vi "FileStream_Create.vi"(7 "mode [OpenOrCreate]":i32(ring)=4 items=["CreateNew"=1, "Create"=2, "Open"=3, "OpenOrCreate"=4, "Truncate"=5, "Append"=6], 8 "error in (no error)":errorcluster, 11 "FilePath":path) -> (0 "error out":errorcluster, 3 "FileStream":refnum<k24>)   [LabVIEW 2018, in "LabVIEWHTTPClient_NET.lvlib" / "HttpContent.lvclass"]
uses:
  HttpContent.lvclass
  Types/HttpNet_error_enum.ctl
  LabVIEWHTTPClient_NET/LabVIEWHTTPClient_NET.lvlib
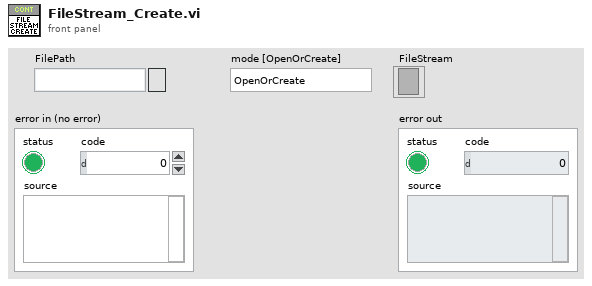
[diagram p1: front panel]
types:
  T1 = typedef "LabVIEWHTTPClient_NET.lvlib/HttpNet_error_enum.ctl" = enum16{"REST method is not available", "URL cannot be blank", "Output filepath cannot be empty", "Input filepath cannot be empty", "Internal .NET error %s", "Output filepath cannot be directory", "Download Task no longer exists"}
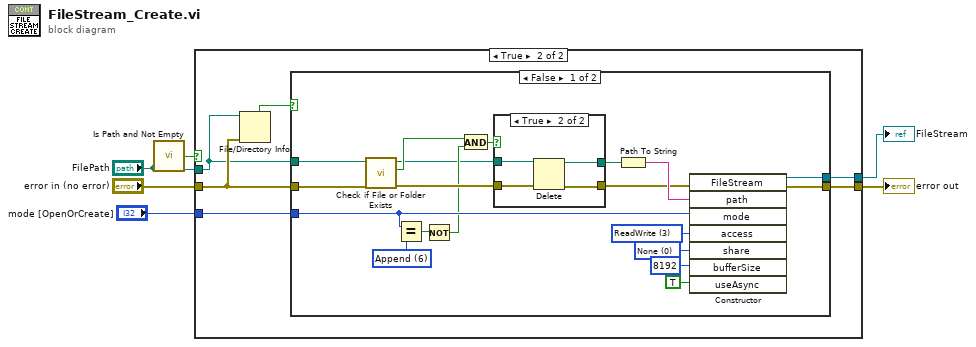
[diagram p0: block diagram]
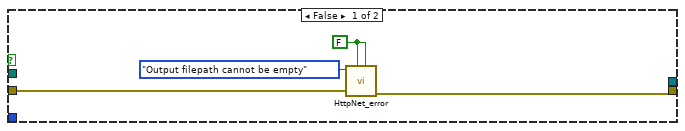
[diagram p2: hidden frame]
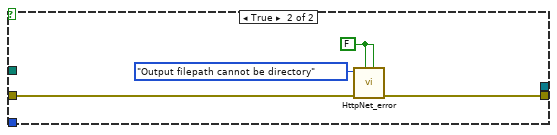
[diagram p4: hidden frame]
diagram:
  n1 = call <vilib>:"Is Path and Not Empty.vi"("path"="FilePath") -> ("Is Path and Not Empty?"=w2:bool)  [unwired: 4 in]
  n2 = case shown="True" w2 {
    tunnel: "error in (no error)" -> [w10 w13]
    tunnel: [w9 w16] -> w5
    tunnel: [_ w15] -> w4
    tunnel: "FilePath" -> [_ w12]
    tunnel: "mode [OpenOrCreate]" -> [_ w14]
    frame False {
      w7 = FALSE ("ShowCallChain [T]")
      n3 = call "HttpNet_error.vi"("ShowCallChain [T]"=w7, "OverrideExistingErrors [T]"=w7, "Error In"=w10, "Error"=HttpNet_error_enum."Output filepath cannot be empty") -> ("Error Out"=w9:errorcluster)  [unwired: 7 in]
    }
    frame True {
      n4 = File/Directory Info(path=w12, error in=w13) -> (directory=w11:bool)  [unwired: 6 out]
      n5 = case shown="False" w11 {
        tunnel: [w32 w42] -> w16
        tunnel: [w31 _] -> w15
        tunnel: w14 -> [w27 _]
        tunnel: w13 -> [w19 w43]
        tunnel: w12 -> [w18 _]
        frame False {
          w26 = 6 items=["CreateNew"=1, "Create"=2, "Open"=3, "OpenOrCreate"=4, "Truncate"=5, "Append"=6] ("mode")
          w33 = 0 items=["None"=0, "Read"=1, "Write"=2, "ReadWrite"=3, "Delete"=4, "Inheritable"=16] ("share")
          w29 = 3 items=["Read"=1, "Write"=2, "ReadWrite"=3] ("access")
          n6 = call <vilib>:"Check if File or Folder Exists.vi"("error in (no error)"=w19, "path"=w18) -> ("error out"=w28:errorcluster, "file or folder exists?"=w23:bool, "dup path"=w21:path)  [unwired: 7 in]
          n7 = Equal?(x=w27, y=w26) -> (x = y?=w25:bool)
          n8 = Not(x=w25) -> (.not. x?=w24:bool)
          n9 = And(x=w23, y=w24) -> (x .and. y?=w22:bool)
          n10 = case shown="True" w22 {
            tunnel: w28 -> [w36 w41]
            tunnel: w21 -> [w37 w40]
            tunnel: [w37 w39] -> w20
            tunnel: [w36 w38] -> w17
            frame False {
            }
            frame True {
              n11 = Delete(path (use dialog)=w40, error in=w41) -> (deleted path=w39:path, error out=w38:errorcluster)  [unwired: 3 in, 1 out]
            }
          }
          n12 = Path To String(path=w20) -> (string=w30:string)
          n13 = constructor class="FileStream"(error in=w17, "path"=w30, "mode"=w27, "access"=w29, "share"=w33, "bufferSize"=8192, "useAsync"=TRUE) -> (reference out=w31:refnum<k24>, error out=w32:errorcluster)  [unwired: 2 in, 7 out]
        }
        frame True {
          w44 = FALSE ("ShowCallChain [T]")
          n14 = call "HttpNet_error.vi"("ShowCallChain [T]"=w44, "OverrideExistingErrors [T]"=w44, "Error In"=w43, "Error"=HttpNet_error_enum."Output filepath cannot be directory") -> ("Error Out"=w42:errorcluster)  [unwired: 7 in]
        }
      }
    }
  }
  "error out" <- w5
  "FileStream" <- w4
